vi "SaveVI.vi"(8 "error in (no error)":errorcluster, 9 "Indicator":string[][](array[string]), 10 "Controls":string[][](array[string]), 11 "Data":string[](array[string])) -> (0 "error out":errorcluster, 2 "status":bool, 3 "VI out":refnum<vi>)   [LabVIEW 2023, in "update vi properties.lvlib"]
uses:
  update vi properties.lvlib
panel:
  # "Connector Pane"
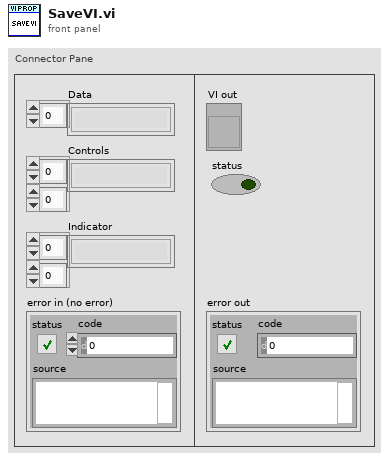
[diagram p1: front panel]
types:
  T1 = enum32{"invalid VI type", "Standard VI", "Control VI", "Global VI", "Polymorphic VI", "Configuration VI", "SubSystem", "Facade VI", "Method VI", "Statechart Diagram VI"}
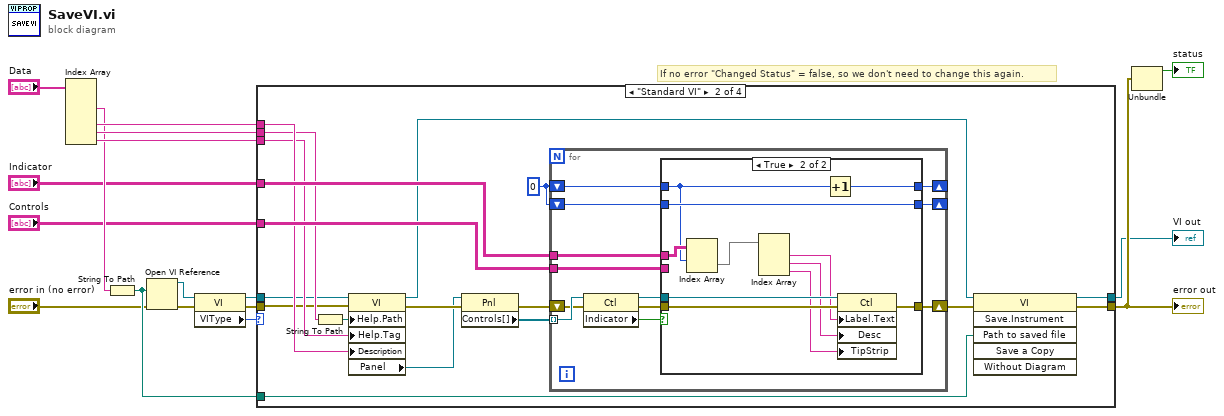
[diagram p0: block diagram]
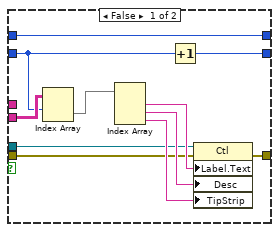
[diagram p3: hidden frame]
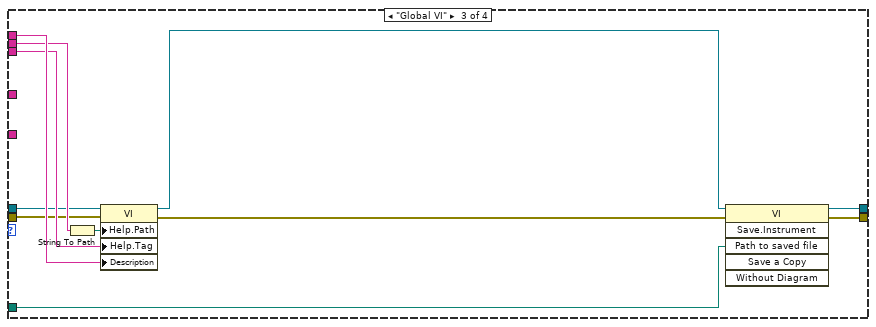
[diagram p4: hidden frame]
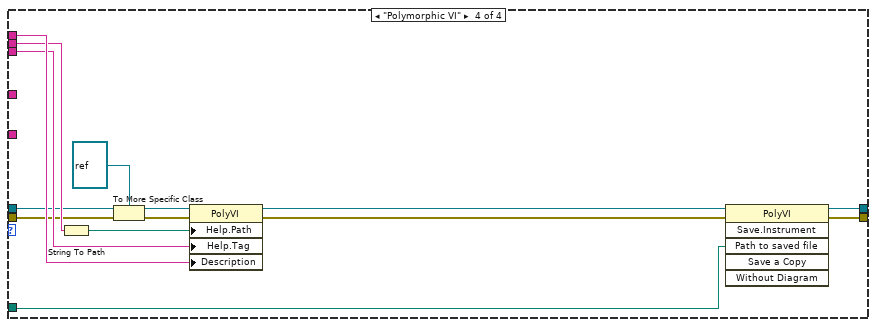
[diagram p5: hidden frame]
diagram:
  # "If no error \"Changed Status\" = false, so we don't need to change this again."
  n1 = Index Array(array="Data") -> (element #2=w5:string, element #4=w6:string, element #5=w8:string, element #6=w7:string)  [unwired: 6 in, 2 out]
  n2 = String To Path(string=w5) -> (path=w9:path)
  n3 = Open VI Reference(vi path=w9, error in (no error)="error in (no error)") -> (vi reference=w10:refnum<vi>, error out=w13:errorcluster)  [unwired: 4 in]
  n4 = property class="VI"(reference=w10, error in=w13) -> (reference out=w11:refnum<vi>, error out=w12:errorcluster, "VIType"=w14:T1)
  n5 = case shown="\"Standard VI\"" w14 {
    tunnel: [w18 w37 w82 w96] -> w15
    tunnel: [w19 w36 w81 w95] -> w16
    tunnel: "Indicator" -> [_ w35 _ _]
    tunnel: "Controls" -> [_ w34 _ _]
    tunnel: w11 -> [w18 w21 w73 w88]
    tunnel: w12 -> [w19 w20 w72 w87]
    tunnel: w6 -> [_ w33 w80 w94]
    tunnel: w7 -> [_ w32 w79 w93]
    tunnel: w8 -> [_ w30 w77 w91]
    tunnel: w9 -> [_ w29 w76 w90]
    frame "invalid VI type", Default {
    }
    frame "Standard VI" {
      w22 = 0
      n6 = String To Path(string=w30) -> (path=w31:path)
      n7 = property class="VI"(reference=w21, error in=w20, "Help.Path"=w31, "Help.Tag"=w32, "Description"=w33) -> (reference out=w25:refnum<vi>, error out=w28:errorcluster, "Panel"=w27:refnum<vi>)
      n8 = property class="Pnl"(reference=w27, error in=w28) -> (error out=w23:errorcluster, "Controls[]"=w24:refnum<vi>[])  [unwired: 1 out]
      n9 = for {
        tunnel: w24 -> [w49] mode=indexing
        shift-right: [w38] -> w26
        shift-left: w23 -> [w48]
        tunnel: w35 -> [w41]
        tunnel: w34 -> [w40]
        shift-right: [w43] -> _
        shift-left: w22 -> [w45]
        shift-right: [w42] -> _
        shift-left: w22 -> [w44]
        n10 = property class="Ctl"(reference=w49, error in=w48) -> (reference out=w39:refnum<vi>, error out=w46:errorcluster, "Indicator"=w47:bool)
        n11 = case shown="True" w47 {
          tunnel: w46 -> [w51 w65]
          tunnel: w45 -> [w59 w68]
          tunnel: w44 -> [w50 w70]
          tunnel: [w59 w71] -> w43
          tunnel: [w60 w70] -> w42
          tunnel: w41 -> [_ w69]
          tunnel: w40 -> [w54 _]
          tunnel: w39 -> [w52 w66]
          tunnel: [w55 w64] -> w38
          frame False {
            n12 = Index Array(array=w54, index (row)=w50) -> (element=w58:string[])  [unwired: 1 in]
            n13 = Index Array(array=w58) -> (element #1=w57:string, element #2=w56:string, element #3=w53:string)  [unwired: 3 in]
            n14 = Increment(x=w50) -> (x+1=w60:i32)
            n15 = property class="Ctl"(reference=w52, error in=w51, "Label.Text"=w57, "Desc"=w56, "TipStrip"=w53) -> (error out=w55:errorcluster)  [unwired: 1 out]
          }
          frame True {
            n16 = Index Array(array=w69, index (row)=w68) -> (element=w67:string[])  [unwired: 1 in]
            n17 = Index Array(array=w67) -> (element #1=w63:string, element #2=w62:string, element #3=w61:string)  [unwired: 3 in]
            n18 = Increment(x=w68) -> (x+1=w71:i32)
            n19 = property class="Ctl"(reference=w66, error in=w65, "Label.Text"=w63, "Desc"=w62, "TipStrip"=w61) -> (error out=w64:errorcluster)  [unwired: 1 out]
          }
        }
      }
      n20 = invoke class="VI" method="Save.Instrument"(reference=w25, error in=w26, "Path to saved file"=w29) -> (reference out=w37:refnum<vi>, error out=w36:errorcluster)  [unwired: 3 in, 4 out]
    }
    frame "Global VI" {
      n21 = String To Path(string=w77) -> (path=w78:path)
      n22 = property class="VI"(reference=w73, error in=w72, "Help.Path"=w78, "Help.Tag"=w79, "Description"=w80) -> (reference out=w74:refnum<vi>, error out=w75:errorcluster)
      n23 = invoke class="VI" method="Save.Instrument"(reference=w74, error in=w75, "Path to saved file"=w76) -> (reference out=w82:refnum<vi>, error out=w81:errorcluster)  [unwired: 3 in, 4 out]
    }
    frame "Polymorphic VI" {
      n24 = String To Path(string=w91) -> (path=w92:path)
      n25 = To More Specific Class(target class=refnum<vi> refnum, reference=w88, error in=w87) -> (specific class reference=w86:refnum<vi>, error out=w85:errorcluster)
      n26 = property class="PolyVI"(reference=w86, error in=w85, "Help.Path"=w92, "Help.Tag"=w93, "Description"=w94) -> (reference out=w84:refnum<vi>, error out=w83:errorcluster)
      n27 = invoke class="PolyVI" method="Save.Instrument"(reference=w84, error in=w83, "Path to saved file"=w90) -> (reference out=w96:refnum<vi>, error out=w95:errorcluster)  [unwired: 3 in, 4 out]
    }
  }
  "error out" <- w16
  "VI out" <- w15
  n28 = Unbundle(w16) -> ("status"=→"status":bool)  [unwired: 2 out]
